vi "MALT23T_002_OneCommand_AllOn.vi"   [LabVIEW 2018]
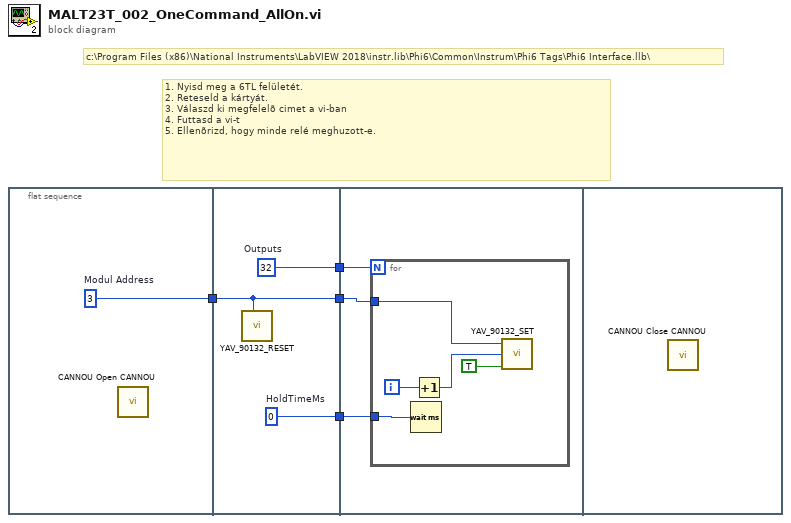
[diagram p0: block diagram]
diagram:
  # "1. Nyisd meg a 6TL felületét.\n2. Reteseld a kártyát.\n3. Válaszd ki megfelelõ cimet a vi-ban\n4. Futtasd a vi-t\n5. Ellenõrizd, hogy minde relé meghuzott-e."
  # "c:\\Program Files (x86)\\National Instruments\\LabVIEW 2018\\instr.lib\\Phi6\\Common\\Instrum\\Phi6 Tags\\Phi6 Interface.llb\\"
  n1 = flat-sequence {
    tunnel: [w5] -> w3
    tunnel: [w8] -> w4
    tunnel: w3 -> [w8]
    tunnel: [w7] -> w2
    tunnel: [w6] -> w1
    tunnel: w4 -> [w11]
    tunnel: w2 -> [w10]
    tunnel: w1 -> [w9]
    frame #0 {
      w5 = u8 3  # Modul Address
      n2 = call <instrlib>:"CANNOU Open CANNOU.vi"() -> ()  [unwired: 6 in, 2 out]
    }
    frame #1 {
      w6 = 0  # HoldTimeMs
      w7 = 32  # Outputs
      n3 = call "YAV_90132_RESET.vi"("Address"=w8) -> ()  [unwired: 4 in, 1 out]
    }
    frame #2 {
      n4 = for {
        N: w10 -> [_]
        tunnel: w11 -> [w12]
        tunnel: w9 -> [w13]
        i -> [w15]
        n5 = Wait (ms)(milliseconds to wait=w13) -> ()  [unwired: 1 out]
        n6 = Increment(x=w15) -> (x+1=w14:i32)
        n7 = call "YAV_90132_SET.vi"("Address"=w12, "Relay Num"=w14, "State"=TRUE) -> ()  [unwired: 2 in, 1 out]
      }
    }
    frame #3 {
      n8 = call <instrlib>:"CANNOU Close CANNOU.vi"() -> ()  [unwired: 7 in, 1 out]
    }
  }
